vi "IMAQ Stack to 1D Array.vi"(8 "error in":errorcluster, 10 "Number of threads":i32, 11 "IMAQ Image Array":T1[](array[typedef])) -> (0 "error out":errorcluster, 3 "Pointer out":u64)   [LabVIEW 2012, in "KLB.lvlib"]
doc: "IMAQ Image Stack to 1D Array\n\nUses LabVIEW memory manager functions to quickly convert a stack of images into a 1D array. The result is given as a pointer to the 1D array.\n\nWill not function for stacks larger then 4GB."
uses:
  KLB.lvlib
  <vilib>/vision/Image Controls.llb/IMAQ Image.ctl
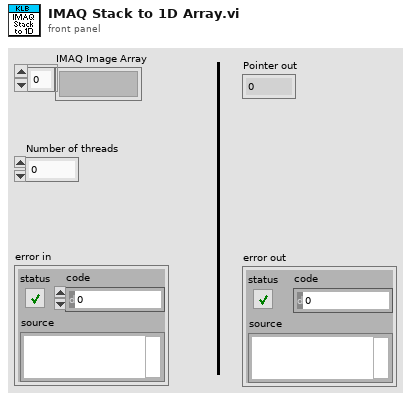
[diagram p1: front panel]
types:
  T1 = typedef "IMAQ Image.ctl" = refnum<image>
  T2 = enum32{"Map Pixel Pointer", "Unmap Pixel Pointer", "Get Pixels Infos"}
  T3 = typedef "Image Type" = u32
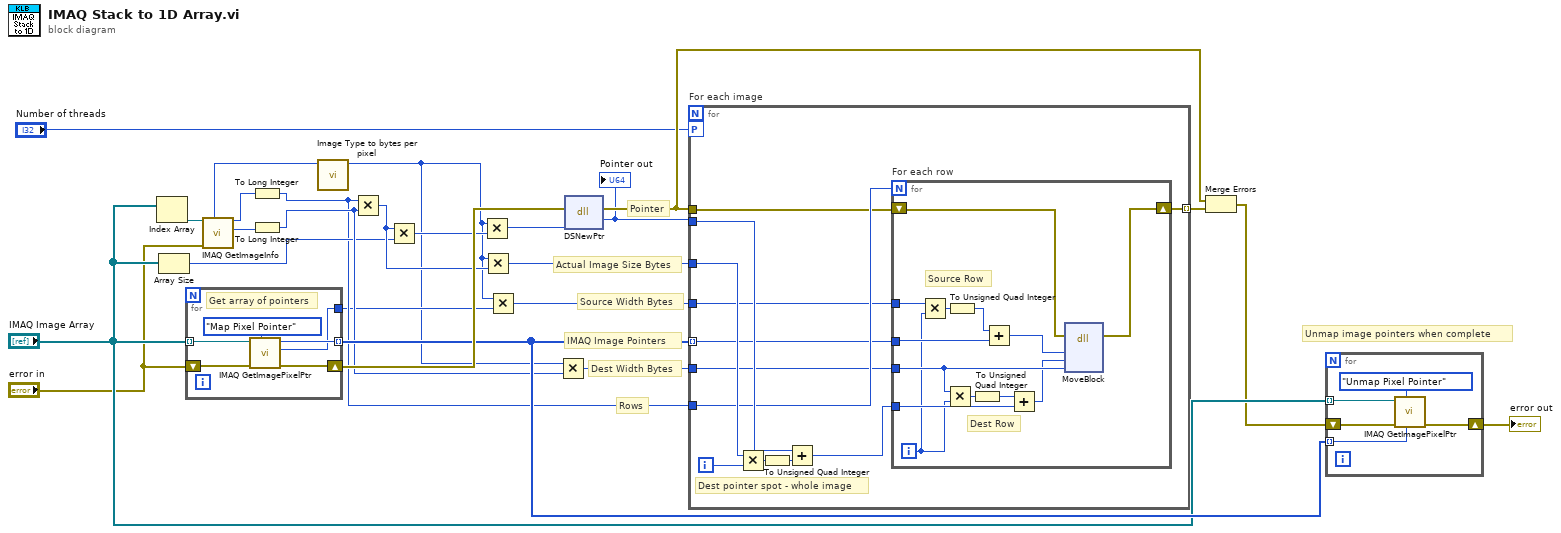
[diagram p0: block diagram]
diagram:
  # "Unmap image pointers when complete"
  # "Pointer"
  # "Rows"
  # "Dest Width Bytes"
  # "Source Width Bytes"
  # "Actual Image Size Bytes"
  # "IMAQ Image Pointers"
  n1 = Index Array(array="IMAQ Image Array") -> (element=w20:T1)  [unwired: 1 in]
  n2 = Array Size(array="IMAQ Image Array") -> (size(s)=w8:i32)
  n3 = for {
    tunnel: "IMAQ Image Array" -> [w27] mode=indexing
    tunnel: [w30] -> w23 mode=indexing
    shift-right: [w28] -> w24
    shift-left: "error in" -> [w29]
    tunnel: [w26] -> w5
    # "Get array of pointers"
    n4 = call "IMAQ GetImagePixelPtr"("Function"=T2."Map Pixel Pointer", "error in (no error)"=w29, "Image"=w27) -> ("error out"=w28:errorcluster, "LineWidth(Pixels)"=w26:i32, "Pixel Pointer out"=w30:u64)  [unwired: 3 in, 3 out]
  }
  n5 = call "IMAQ GetImageInfo"("error in (no error)"="error in", "Image"=w20) -> ("Y Resolution"=w18:i32, "X Resolution"=w19:i32, "Image Type"=w16:T3)  [unwired: 2 in, 5 out]
  n6 = To Long Integer(number=w19) -> (32bit integer=w7:i32)
  n7 = To Long Integer(number=w18) -> (32bit integer=w10:i32)
  n8 = call "Image Type to bytes per pixel.vi"("Image Type"=w16) -> ("Bytes per Pixel"=w4:u32)  [unwired: 10 in]
  n9 = Multiply(x=w7, y=w10) -> (x*y=w12:i32)
  n10 = Multiply(x=w12, y=w8) -> (x*y=w15:i32)
  n11 = Multiply(x=w4, y=w15) -> (x*y=w14:u32)
  n12 = Multiply(x=w4, y=w12) -> (x*y=w11:u32)
  n13 = Multiply(x=w4, y=w5) -> (x*y=w6:u32)
  n14 = Multiply(x=w4, y=w10) -> (x*y=w9:u32)
  n15 = dll-call lib="LabVIEW" fn="DSNewPtr"(error in=w24, "Size"=w14) -> (error out=w25:errorcluster, "Pointer"=w13:u64)  [unwired: 3 in, 1 out]
  "Pointer out" <- w13
  n16 = for "For each image" {
    tunnel: w23 -> [w36] mode=indexing
    tunnel: w13 -> [w41]
    tunnel: w11 -> [w42]
    workers-P: "Number of threads" -> [_]
    tunnel: w6 -> [w35]
    tunnel: w9 -> [w37]
    tunnel: w7 -> [w38]
    tunnel: w25 -> [w32]
    tunnel: [w33] -> w3 mode=indexing
    i -> [w43]
    # "Dest pointer spot - whole image"
    n17 = Multiply(x=w42, y=w43) -> (x*y=w40:u32)
    n18 = To Unsigned Quad Integer(1:w40) -> (0:w39:u64)
    n19 = Add(x=w41, y=w39) -> (x+y=w34:u64)
    n20 = for "For each row" {
      N: w38 -> [_]
      tunnel: w37 -> [w48]
      tunnel: w36 -> [w55]
      tunnel: w35 -> [w54]
      tunnel: w34 -> [w56]
      shift-right: [w44] -> w33
      shift-left: w32 -> [w45]
      i -> [w47]
      # "Dest Row"
      # "Source Row"
      n21 = Multiply(x=w54, y=w47) -> (x*y=w51:u32)
      n22 = Multiply(x=w48, y=w47) -> (x*y=w49:u32)
      n23 = To Unsigned Quad Integer(1:w51) -> (0:w52:u64)
      n24 = To Unsigned Quad Integer(1:w49) -> (0:w50:u64)
      n25 = Add(x=w52, y=w55) -> (x+y=w53:u64)
      n26 = Add(x=w50, y=w56) -> (x+y=w46:u64)
      n27 = dll-call lib="LabVIEW" fn="MoveBlock"(error in=w45, "Source"=w53, "Destination"=w46, "Size"=w48) -> (error out=w44:errorcluster)  [unwired: 6 in, 1 out]
    }
  }
  n28 = Merge Errors(w25, w3) -> (w21:errorcluster)
  n29 = for {
    shift-right: [w59] -> w1
    shift-left: w21 -> [w60]
    tunnel: "IMAQ Image Array" -> [w58] mode=indexing
    tunnel: w23 -> [w57] mode=indexing
    n30 = call "IMAQ GetImagePixelPtr"("Pixel Pointer in"=w57, "Function"=T2."Unmap Pixel Pointer", "error in (no error)"=w60, "Image"=w58) -> ("error out"=w59:errorcluster)  [unwired: 2 in, 5 out]
  }
  "error out" <- w1
